vi "coerce exposure to available increment.vi"(6 "desired exposure":dbl, 9 "Increment":dbl, 10 "Min":dbl, 11 "Max":dbl) -> (3 "closest available exposure":dbl)   [LabVIEW 2020]
panel:
  out "floor(x/y)":dbl
  out "x-y*floor(x/y)":dbl
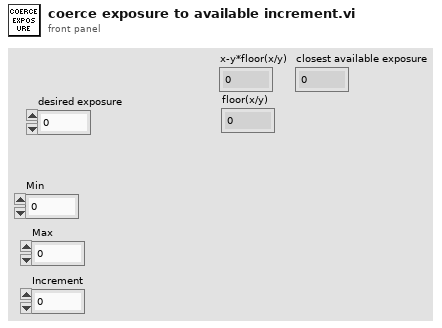
[diagram p1: front panel]
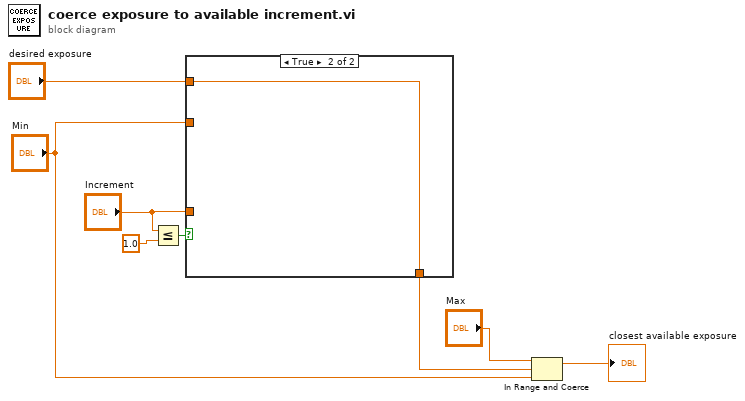
[diagram p0: block diagram]
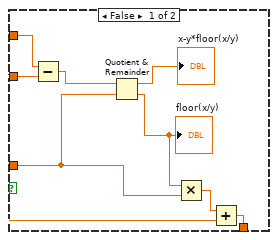
[diagram p2: hidden frame]
diagram:
  n1 = Less Or Equal?(x="Increment", y=1.0) -> (x <= y?=w1:bool)
  n2 = case shown="True" w1 {
    tunnel: "desired exposure" -> [w16 w17]
    tunnel: [w11 w17] -> w6
    tunnel: "Min" -> [w10 _]
    tunnel: "Increment" -> [w9 _]
    frame False {
      n3 = Subtract(x=w16, y=w10) -> (x-y=w15:dbl)
      n4 = Quotient & Remainder(x=w15, y=w9) -> (x-y*floor(x/y)=→"x-y*floor(x/y)":dbl, floor(x/y)=w13:dbl)
      "floor(x/y)" <- w13
      n5 = Multiply(x=w13, y=w9) -> (x*y=w12:dbl)
      n6 = Add(x=w12, y=w10) -> (x+y=w11:dbl)
    }
    frame True {
    }
  }
  n7 = In Range and Coerce(upper limit="Max", x=w6, lower limit="Min") -> (coerced(x)=→"closest available exposure":dbl)  [unwired: 1 out]
